vi "midiInGetErrorTextA.vi"(8 "error in":errorcluster, 11 "Error Code":i32) -> (0 "error out":errorcluster)   [LabVIEW 2020, in "midi.lvclass"]
doc: "The midiOutGetErrorText function retrieves a textual description for an error identified by the specified error code."
uses:
  midi.lvclass
  midi.lvclass/midi.ctl
  winmm.dll
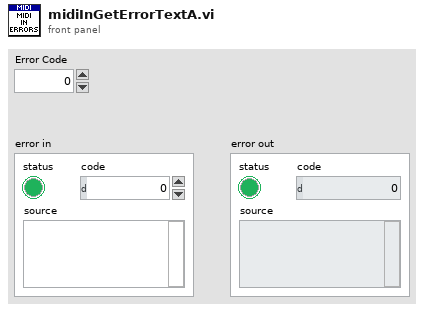
[diagram p1: front panel]
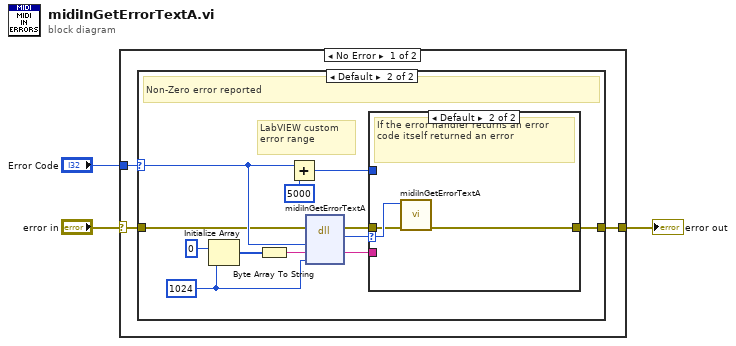
[diagram p0: block diagram]
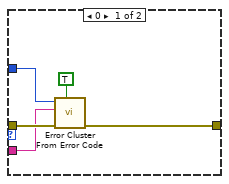
[diagram p3: hidden frame]
diagram:
  n1 = case shown="No Error" "error in" {
    selector: "error in" -> [w5 w28]
    tunnel: "Error Code" -> [w6 _]
    tunnel: [w4 w28] -> w1
    frame No Error {
      n2 = case shown="Default" w6 {
        selector: w6 -> [_ w18]
        tunnel: w5 -> [w7 w12]
        tunnel: [w7 w8] -> w4
        frame 0 {
          # "0 = No Error was returned"
        }
        frame Default {
          w14 = 1024 ("dimension size")
          # "LabVIEW custom error range"
          # "Non-Zero error reported"
          n3 = Initialize Array(u8 0, w14) -> (w16:u8[])
          n4 = Byte Array To String(unsigned byte array=w16) -> (string=w15:string)
          n5 = Add(x=w18, y=5000) -> (x+y=w9:i32)
          n6 = dll-call lib="winmm.dll" fn="midiInGetErrorTextA"(error in=w12, "mmrError"=w18, "pszText"=w15, "cchText"=w14) -> (error out=w11:errorcluster, "error code"=w13:i32, "pszText"=w10:string)  [unwired: 4 in, 1 out]
          n7 = case shown="Default" w13 {
            selector: w13 -> [_ w27]
            tunnel: w11 -> [w23 w26]
            tunnel: w10 -> [w22 _]
            tunnel: w9 -> [w21 _]
            tunnel: [w20 w25] -> w8
            frame 0 {
              n8 = call <vilib>:"Error Cluster From Error Code.vi"("show call chain? (False)"=TRUE, "error in (no error)"=w23, "error message (\"\")"=w22, "error code (0)"=w21) -> ("error out"=w20:errorcluster)  [unwired: 5 in]
            }
            frame Default {
              # "If the error handler returns an error code itself returned an error"
              n9 = call "midiInGetErrorTextA.vi"("error in"=w26, "Error Code"=w27) -> ("error out"=w25:errorcluster)  [unwired: 9 in]
            }
          }
        }
      }
    }
    frame Error {
    }
  }
  "error out" <- w1
